vi "schleife fluss.vi"() -> ()   [LabVIEW 2010]
panel:
  out "Aktuelle Zeit":timestamp
  out "Durchlauf Nr.":i32
  in  "?":bool
  out "Wert des Zustandes \"i\"":i32
  in  "Werte der Zustände":i32[](array[numeric])=[1, 3, 5, 2]
  in  "Längen der Zustände (s)":i32[](array[numeric])=[1, 3, 5, 2]
  out "Länge des Zustandes \"i\" (s)":i32
  out "Anzahl der Zustände":i32
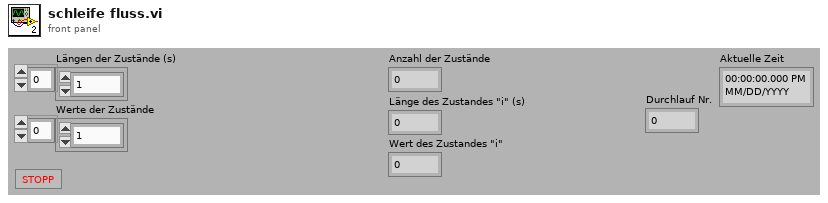
[diagram p1: front panel]
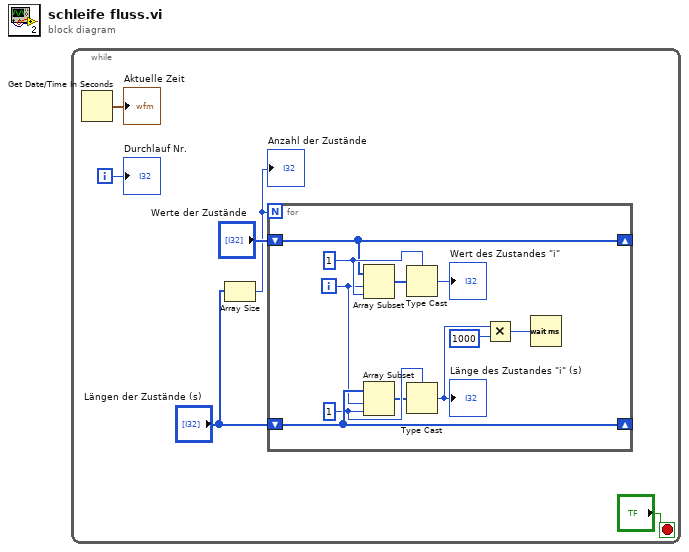
[diagram p0: block diagram]
diagram:
  n1 = while {
    i -> [w2]
    stop <- "?" stop-if-true
    n2 = Get Date/Time In Seconds() -> (seconds since 1Jan1904=→"Aktuelle Zeit":timestamp)
    n3 = Array Size(array="Längen der Zustände (s)") -> (size(s)=w4:i32)
    "Anzahl der Zustände" <- w4
    n4 = for {
      N: w4 -> [_]
      shift-right: [w16] -> _
      shift-left: "Längen der Zustände (s)" -> [w16]
      shift-right: [w7] -> _
      shift-left: "Werte der Zustände" -> [w7]
      i -> [w8]
      w11 = 1 ("Länge")
      w15 = 1 ("Länge")
      n5 = Array Subset(array=w7, index=w8, length=w11) -> (w10:i32[])
      n6 = Array Subset(array=w16, index=w8, length=w15) -> (w14:i32[])
      n7 = Type Cast(type=w11, x=w10) -> (*(type *) &x=→"Wert des Zustandes \"i\"":i32)
      n8 = Type Cast(type=w15, x=w14) -> (*(type *) &x=w13:i32)
      "Länge des Zustandes \"i\" (s)" <- w13
      n9 = Multiply(x=w13, y=1000) -> (x*y=w12:i32)
      n10 = Wait (ms)(milliseconds to wait=w12) -> ()  [unwired: 1 out]
    }
    "Durchlauf Nr." <- w2
  }
